vi "Supervisor MATLAB Write Client.vi"() -> ()   [LabVIEW 2017]
uses:
  <vilib>/OPCUA/controls/Write Status.ctl
  <vilib>/OPCUA/controls/NodeId.ctl
  <vilib>/OPCUA/client/Multiple Write Bool Array.vi
  <vilib>/OPCUA/NI OPC UA Client.lvlib
panel:
  in  "Stop MATLAB Control":bool
  in  "Node Status":T1 items=["Good"=0, "Uncertain_InitialValue"=1083310080, "Uncertain_LastUsableValue"=1083179008, "Uncertain_SensorNotAccurate"=1083375616, "Uncertain_EngineeringUnitsExceeded"=1083441152, "Bad_NoCommunication"=2150694912, "Bad_NotReadable"=2151284736, "Bad_NotWritable"=2151350272, "Bad_OutOfRange"=2151415808, "Bad_WaitingForInitialData"=2150760448]
  in  "Time Stamp":timestamp
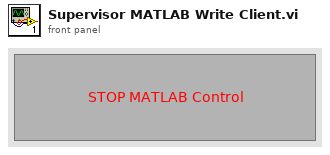
[diagram p1: front panel]
types:
  T1 = typedef "Write Status.ctl" = u32
  T2 = cluster{"message mode":enum16{"None", "Sign", "Sign and Encrypt"}, "security":enum16{"Basic256", "Basic128Rsa15"}}
  T3 = typedef "OPC UA Client Refnum.ctl" = refnum<k21>
  T4 = typedef "NodeId.ctl" = string
  T5 = cluster{"node ID":T4, "value":bool[], "timestamp (current time)":timestamp, "node status":T1}
  T6 = cluster{"node ID":T4, "value":bool[], "timestamp (current time)":timestamp, "node status":T1}[]
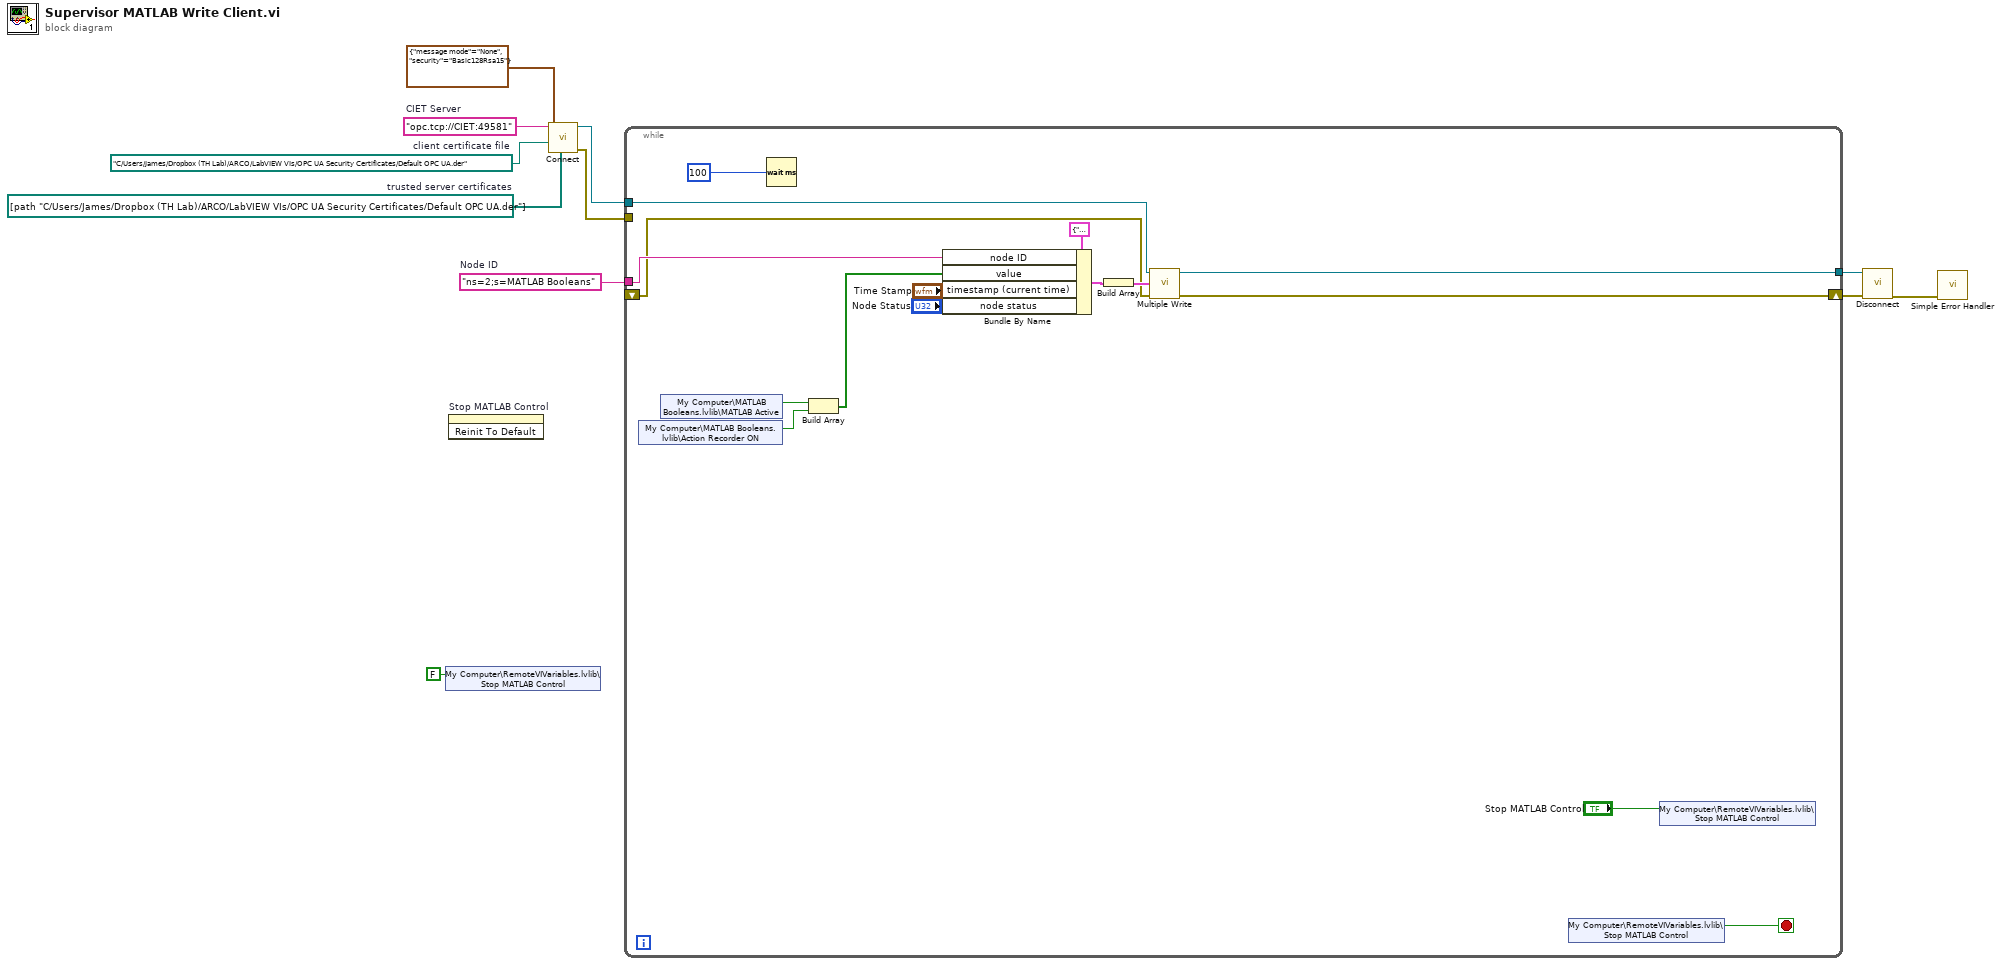
[diagram p0: block diagram]
diagram:
  w7 = "ns=2;s=MATLAB Booleans"  # Node ID
  w8 = path[] [path "C:/Users/James/Dropbox (TH Lab)/ARCO/LabVIEW VIs/OPC UA Security Certificates/Default OPC UA.der"]  # trusted server certificates
  w9 = path "C:/Users/James/Dropbox (TH Lab)/ARCO/LabVIEW VIs/OPC UA Security Certificates/Default OPC UA.der"  # client certificate file
  w11 = "opc.tcp://CIET:49581"  # CIET Server
  n1 = shared-variable "My Computer\\RemoteVIVariables.lvlib\\Stop MATLAB Control"(FALSE ("Stop MATLAB Control")) -> ()  [unwired: 1 in, 1 out]
  n2 = invoke on="Stop MATLAB Control" class="Bool (strict)" method="Reinit To Default"() -> ()  [unwired: 3 in, 3 out]
  n3 = call <vilib>:"Connect.vi"("trusted server certificates"=w8, "client certificate file"=w9, "security policy"=T2 {"message mode"=enum."None", "security"=enum."Basic128Rsa15"}, "server endpoint URL"=w11) -> ("error out"=w6:errorcluster, "OPC UA client refnum out"=w5:T3)  [unwired: 5 in, 1 out]
  n4 = while {
    tunnel: w7 -> [w23]
    tunnel: w6 -> [_]
    tunnel: w5 -> [w17]
    tunnel: [w16] -> w3
    shift-right: [w15] -> w2
    shift-left: _ -> [w14]
    stop <- w12 stop-if-true
    n5 = shared-variable "My Computer\\MATLAB Booleans.lvlib\\Action Recorder ON"() -> (w25:bool)  [unwired: 1 in, 1 out]
    n6 = shared-variable "My Computer\\MATLAB Booleans.lvlib\\MATLAB Active"() -> (w26:bool)  [unwired: 1 in, 1 out]
    n7 = Wait (ms)(milliseconds to wait=u32 100) -> ()  [unwired: 1 out]
    n8 = Build Array(w26, w25) -> (w24:bool[])
    n9 = Bundle By Name(cluster=T5 {"node ID"="", "value"=[], "timestamp (current time)"=timestamp(0 s since 1904-01-01), "node status"=0} ("request"), "node ID"=w23, "value"=w24, "timestamp (current time)"="Time Stamp", "node status"="Node Status") -> (w19:T5)
    n10 = Build Array(w19) -> (w18:T6)
    n11 = call-poly <vilib>:"Multiple Write.vi"("error in (no error)"=w14, "requests"=w18, "OPC UA client refnum in"=w17) -> ("error out"=w15:errorcluster, "OPC UA client refnum out"=w16:T3)  [unwired: 5 in, 2 out]
    n12 = shared-variable "My Computer\\RemoteVIVariables.lvlib\\Stop MATLAB Control"() -> (w12:bool)  [unwired: 1 in, 1 out]
    n13 = shared-variable "My Computer\\RemoteVIVariables.lvlib\\Stop MATLAB Control"("Stop MATLAB Control") -> ()  [unwired: 1 in, 1 out]
  }
  n14 = call <vilib>:"Disconnect.vi"("error in (no error)"=w2, "OPC UA client refnum in"=w3) -> ("error out"=w4:errorcluster)  [unwired: 9 in]
  n15 = call <vilib>:"Simple Error Handler.vi"("error in (no error)"=w4) -> ()  [unwired: 4 in, 5 out]
